vi "Compute Roughness Params.vi"(8 "error in (no error)":errorcluster, 11 "Video Cam Processor in":refnum<class "Video Cam Processor.lvclass">) -> (0 "error out":errorcluster, 3 "Video Cam Processor out":refnum<class "Video Cam Processor.lvclass">)   [LabVIEW 2018, in "Video Cam Processor.lvclass"]
uses:
  Video Cam Processor.lvclass
  Video Cam Processor.lvclass/Video Cam Processor.ctl
  801cfc77-0225-4dd6-8cac-499286138bf7.vi
  6ba7fa41-93de-4c8f-8f22-701f1a22bb08.vi
  801cfc77-0225-4dd6-8cac-499286138bf7.vi/ccb2f2df-29a9-4baf-b55c-03840807a134.vi
  Video Frame/Video Frame.lvclass
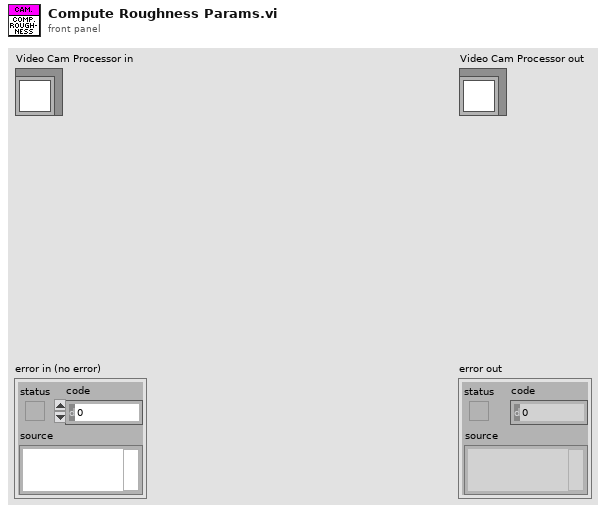
[diagram p1: front panel]
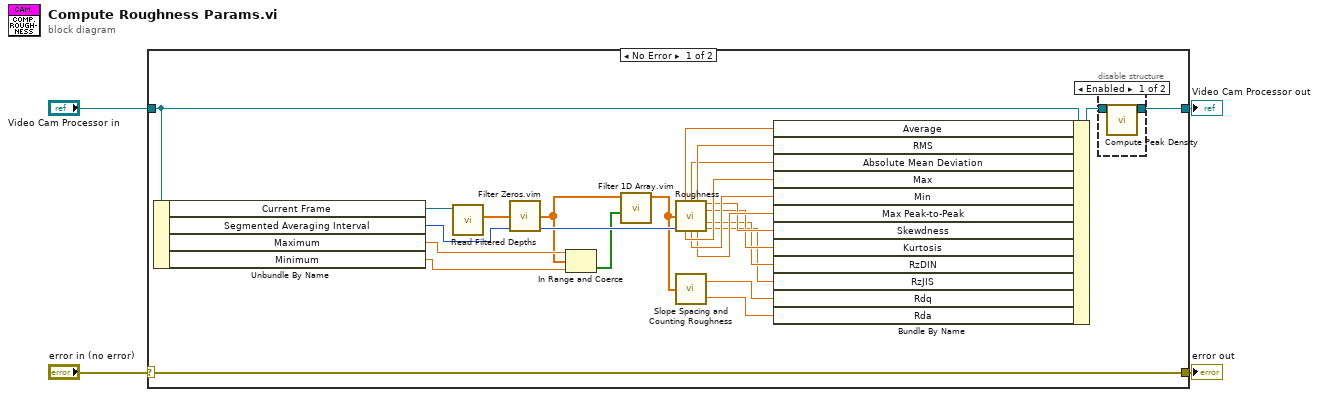
[diagram p0: block diagram]
diagram:
  n1 = case shown="No Error" "error in (no error)" {
    selector: "error in (no error)" -> [w28 w33]
    tunnel: [w28 w33] -> w3
    tunnel: [w12 w32] -> w1
    tunnel: "Video Cam Processor in" -> [w26 w32]
    frame No Error {
      n2 = Unbundle By Name(w26) -> ("Current Frame"=w27:refnum<class "Video Frame.lvclass">, "Segmented Averaging Interval"=w11:i32, "Maximum"=w9:dbl, "Minimum"=w8:dbl)
      n3 = call-dynamic "Read Filtered Depths.vi"("Video Frame in"=w27) -> ("Filtered Depths"=w10:dbl[])  [unwired: 8 in, 2 out]
      n4 = call "Filter Zeros.vim"("Array"=w10) -> ("Array Out"=w7:dbl[])  [unwired: 14 in]
      n5 = In Range and Coerce(upper limit=w9, x=w7, lower limit=w8) -> (In Range?=w6:bool[])  [unwired: 1 out]
      n6 = call "Filter 1D Array.vim"("Boolean Filter"=w6, "Array"=w7) -> ("Array Out"=w5:dbl[])  [unwired: 9 in]
      n7 = call "Roughness.vi"("Data"=w5, "Sub Sampling Interval (10)"=w11) -> ("Mean"=w25:dbl, "Absolute Mean Deviation"=w23:dbl, "RMS"=w24:dbl, "Skewdness"=w19:dbl, "Kurtosis"=w18:dbl, "RzDIN"=w17:dbl, "Max"=w22:dbl, "Min"=w21:dbl, "Max P-P"=w20:dbl, "RzJIS"=w16:dbl)  [unwired: 4 in]
      n8 = call "Slope Spacing and Counting Roughness.vi"("Data"=w5) -> ("Rdq"=w15:dbl, "Rda"=w14:dbl)  [unwired: 4 in]
      n9 = Bundle By Name(cluster=w26, "Average"=w25, "RMS"=w24, "Absolute Mean Deviation"=w23, "Max"=w22, "Min"=w21, "Max Peak-to-Peak"=w20, "Skewdness"=w19, "Kurtosis"=w18, "RzDIN"=w17, "RzJIS"=w16, "Rdq"=w15, "Rda"=w14) -> (w13:refnum<class "Video Cam Processor.lvclass">)
      n10 = disable-structure shown="Enabled" {
        disable-tunnel: w13 -> [w30 w31]
        disable-tunnel: [w29 w31] -> w12
        frame Enabled {
          n11 = call-dynamic "Compute Peak Density.vi"("Video Cam Processor in"=w30) -> ("Video Cam Processor out"=w29:refnum<class "Video Cam Processor.lvclass">)  [unwired: 8 in, 2 out]
        }
        frame Disabled {
        }
      }
    }
    frame Error {
    }
  }
  "error out" <- w3
  "Video Cam Processor out" <- w1
